vi "Filter Bookmarks.vi"(8 "Error In":errorcluster, 11 "All Bookmarks":T2) -> (0 "Error Out":errorcluster, 3 "Eulogy Bookmarks":T1(array[cluster]))   [LabVIEW 2017, in "Graveyard.lvlib"]
doc: "Filters out all bookmarks that are NOT graves"
uses:
  Graveyard.lvlib
  <vilib>/Utility/miscctls.llb/LVBookmarkInfoTypeDef.ctl
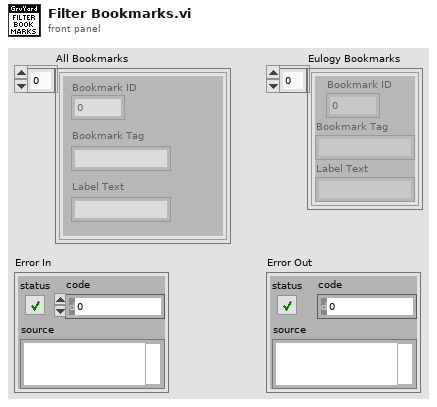
[diagram p1: front panel]
types:
  T1 = cluster{"Bookmark ID":u32, "Bookmark Tag":string, "Label Text":string}[]
  T2 = typedef "LVBookmarkInfoTypeDef.ctl" = cluster{"Bookmark ID":u32, "Bookmark Tag":string, "Label Text":string}[]
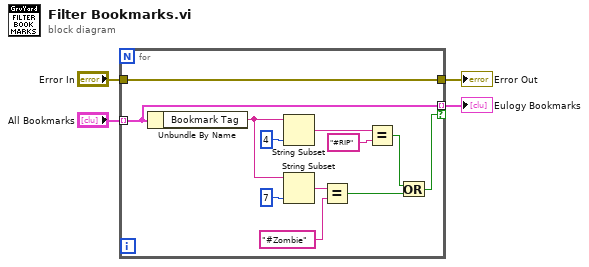
[diagram p0: block diagram]
diagram:
  n1 = for {
    tunnel: "All Bookmarks" -> [w13] mode=indexing
    tunnel: [w13] -> w3 mode=indexing if=w11
    tunnel: "Error In" -> [w12]
    tunnel: [w12] -> w1
    n2 = Unbundle By Name(w13) -> ("Bookmark Tag"=w9:string)
    n3 = String Subset(string=w9, length (rest)=4 ("length (rest)")) -> (substring=w15:string)  [unwired: 1 in]
    n4 = String Subset(string=w9, length (rest)=7 ("length (rest)")) -> (substring=w7:string)  [unwired: 1 in]
    n5 = Equal?(x=w7, y="#Zombie") -> (x = y?=w5:bool)
    n6 = Equal?(x=w15, y="#RIP") -> (x = y?=w10:bool)
    n7 = Or(x=w10, y=w5) -> (x .or. y?=w11:bool)
  }
  "Eulogy Bookmarks" <- w3
  "Error Out" <- w1
